vi "SetAmpControl.vi"(0 "Amplitude Control Cluster":T1={"Amplitude"=-inf, "Min"=-inf, "Max"=-inf, "P"=-inf, "I"=-inf, "Setpoint"=-inf, "Invert Polarity"=-2147483648, "Loop"=FALSE} {"Invert Polarity" items=["[read only]"=-2147483648, "No"=0, "Yes"=1]; "Setpoint" format="%#_g V"; "I" format="%#_g Hz"; "Max" format="%#_g V"; "Min" format="%#_g V"; "Amplitude" format="%#_g V"}, 5 "error in":T3) -> (14 "Output Cluster":T1={"Amplitude"=-inf, "Min"=-inf, "Max"=-inf, "P"=-inf, "I"=-inf, "Setpoint"=-inf, "Invert Polarity"=-2147483648, "Loop"=FALSE} {"Invert Polarity" items=["[read only]"=-2147483648, "No"=0, "Yes"=1]; "Setpoint" format="%#_g V"; "I" format="%#_g Hz"; "Max" format="%#_g V"; "Min" format="%#_g V"; "Amplitude" format="%#_g V"}, 19 "error out":T3)   [LabVIEW 2016]
doc: "Sets all relevant parameters for the operation of an amplitude control:\n- Amplitude in V (float) [0 to 10]\n- Min in kHz (float) [0 to 10]\n- Max in kHz (float) [0 to 10]\n- P (float) [0 to 100]\n- I in mHz (float) [0 to 1000000]\n- Setpoint in V (float) [-10 to 10]\n- Invert Polarity (integer) [0 -- no; 1 -- yes]\nBy passing -Inf (float) or -2147483648 (integer) the corresponding value will be read out."
uses:
  Controls/Amplitude-Control_Parameters.ctl
  Controls/Invert-Polarity_Selection.ctl
  Controls/Error_Out.ctl
  Files_ASC500/DLL/ASC500_RemoteControlV27.dll
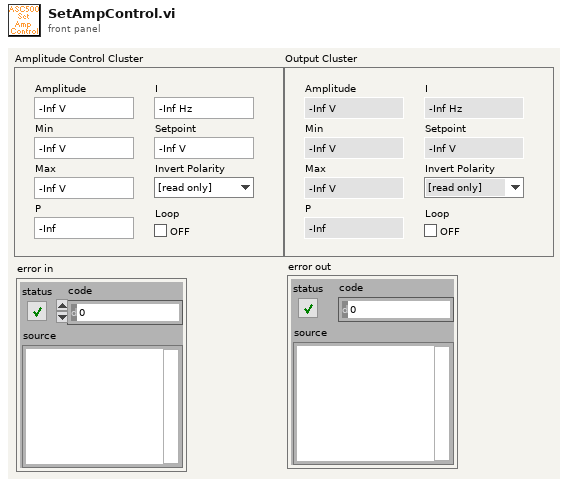
[diagram p1: front panel]
types:
  T1 = typedef "Amplitude-Control_Parameters.ctl" = cluster{"Amplitude":sgl, "Min":sgl, "Max":sgl, "P":sgl, "I":sgl, "Setpoint":sgl, "Invert Polarity":T2, "Loop":bool}
  T2 = typedef "Invert-Polarity_Selection.ctl" = i32
  T3 = typedef "Error_Out.ctl" = errorcluster
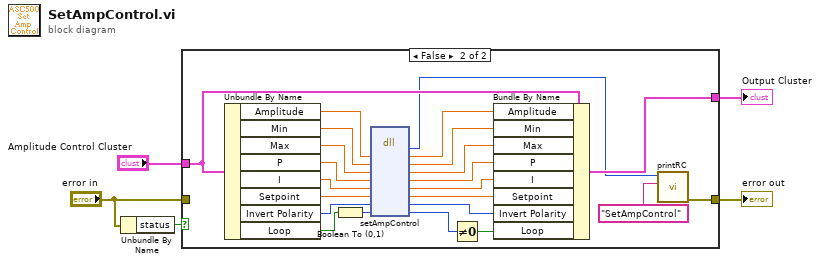
[diagram p0: block diagram]
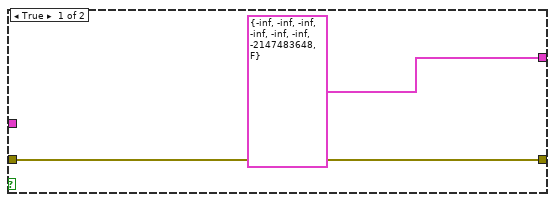
[diagram p2: hidden frame]
diagram:
  n1 = Unbundle By Name("error in") -> ("status"=w5:bool)
  n2 = case shown="False" w5 {
    tunnel: [w6 w15] -> w4
    tunnel: "Amplitude Control Cluster" -> [_ w18]
    tunnel: [T1 {"Amplitude"=-inf, "Min"=-inf, "Max"=-inf, "P"=-inf, "I"=-inf, "Setpoint"=-inf, "Invert Polarity"=-2147483648, "Loop"=FALSE} ("Amplitude Control Cluster") w17] -> w2
    tunnel: "error in" -> [w6 _]
    frame True {
    }
    frame False {
      n3 = Unbundle By Name(w18) -> ("Amplitude"=w25:sgl, "Min"=w26:sgl, "Max"=w27:sgl, "P"=w28:sgl, "I"=w29:sgl, "Setpoint"=w30:sgl, "Invert Polarity"=w16:T2, "Loop"=w11:bool)
      n4 = Boolean To (0,1)(Boolean=w11) -> (0, 1=w10:i16)
      n5 = dll-call lib="G:/SCMOperations/Share/ELE/Produkt Information/ASC500/04 Remote Control/02 development versions/2018Nov06/Files_ASC500/DLL/ASC500_RemoteControlV27.dll" fn="setAmpControl"("Amplitude"=w25, "Min"=w26, "Max"=w27, "P"=w28, "I"=w29, "Setpoint"=w30, "Invert Polarity"=w16, "Loop"=w10) -> ("return type"=w13:i32, "Amplitude"=w24:sgl, "Min"=w19:sgl, "Max"=w20:sgl, "P"=w21:sgl, "I"=w22:sgl, "Setpoint"=w23:sgl, "Invert Polarity"=w12:i32, "Loop"=w8:i32)  [unwired: 3 in, 2 out]
      n6 = Not Equal To 0?(x=w8) -> (x != 0?=w9:bool)
      n7 = Bundle By Name(cluster=w18, "Amplitude"=w24, "Min"=w19, "Max"=w20, "P"=w21, "I"=w22, "Setpoint"=w23, "Invert Polarity"=w12, "Loop"=w9) -> (w17:T1)
      n8 = call "printRC.vi"("additional information"="SetAmpControl", "RC"=w13) -> ("error out"=w15:T3)  [unwired: 9 in]
    }
  }
  "error out" <- w4
  "Output Cluster" <- w2
